vi "Get Steering Type.vi"(8 "error in (no error)":errorcluster, 11 "ackermann steering frame in":refnum<class "NI_Robotics_Ackermann Steering Frame.lvclass">) -> (0 "error out":errorcluster, 2 "steering type":string, 3 "ackermann steering frame out":refnum<class "NI_Robotics_Ackermann Steering Frame.lvclass">)   [LabVIEW 2017, in "NI_Robotics_Ackermann Steering Frame.lvclass"]
uses:
  <vilib>/robotics/Steering/Ackermann Steering Frame/NI_Robotics_Ackermann Steering Frame.lvclass
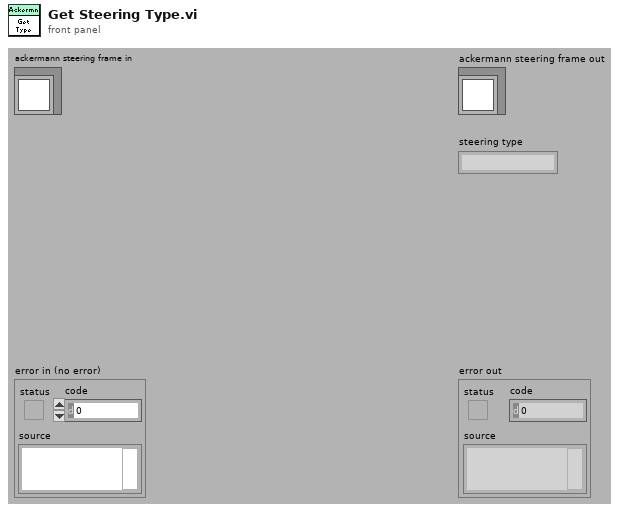
[diagram p1: front panel]
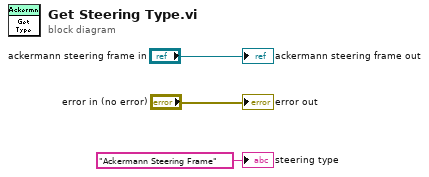
[diagram p0: block diagram]
diagram:
  "error out" <- "error in (no error)"
  "ackermann steering frame out" <- "ackermann steering frame in"
  "steering type" <- "Ackermann Steering Frame" ("Steering Type")
